vi "Parse RS232 Data to Integer.vi"(9 "AML end byte":i32, 10 "AML start byte":i32, 11 "bytes in":string) -> (2 "I32 data":i32, 3 "bytes out":string)   [LabVIEW 2019, in "PGC2D.lvlib"]
uses:
  PGC2D.lvlib
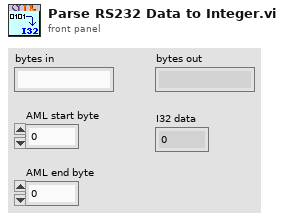
[diagram p1: front panel]
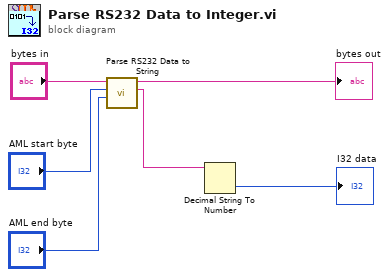
[diagram p0: block diagram]
diagram:
  n1 = call "Parse RS232 Data to String.vi"("AML end byte"="AML end byte", "AML start byte"="AML start byte", "bytes in"="bytes in") -> ("string data"=w2:string, "bytes out"=→"bytes out":string)  [unwired: 7 in]
  n2 = Decimal String To Number(string=w2) -> (number=→"I32 data":i32)  [unwired: 2 in, 1 out]
